vi "Test Get Right Menu on Card Inserted.vi"(8 "error in (no error)":errorcluster, 11 "Test Case In":refnum<class "View Model Test.lvclass">) -> (0 "error out":errorcluster, 3 "Test Case Out":refnum<class "View Model Test.lvclass">)   [LabVIEW 2020, in "View Model Test.lvclass"]
uses:
  View Model Test.lvclass
  View Model Test.lvclass/View Model Test.ctl
  01074fa8-ee8a-411d-bc8b-fc92c4f90959.vi
  ATM View Model/ATM View Model.lvclass
  ATM Controller/State.ctl
  ATM Controller/ATM Controller.lvclass
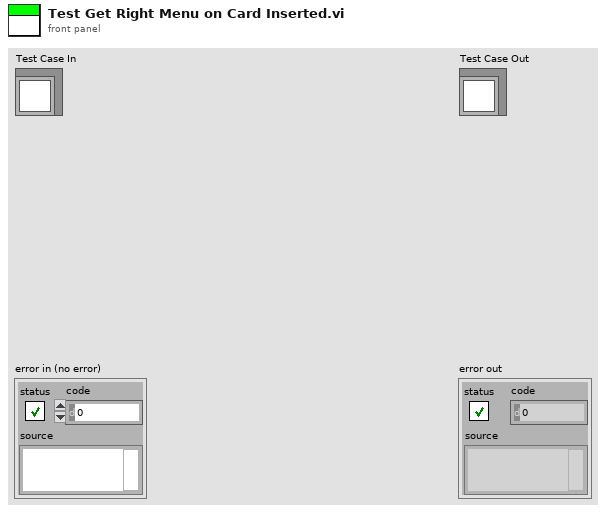
[diagram p1: front panel]
types:
  T1 = cluster{"RFS String":string, "RFS String 2":string, "RFS String 3":string}
  T2 = typedef "ATM Controller.lvclass/State.ctl" = enum16{"Start", "Card Inserted", "Verification Failed", "Verification Succeeded", "Depositing", "Depositing Completed", "Withdrawing", "Withdraw Completed", "Withdraw Failed", "Balance Inquiry", "Terminate"}
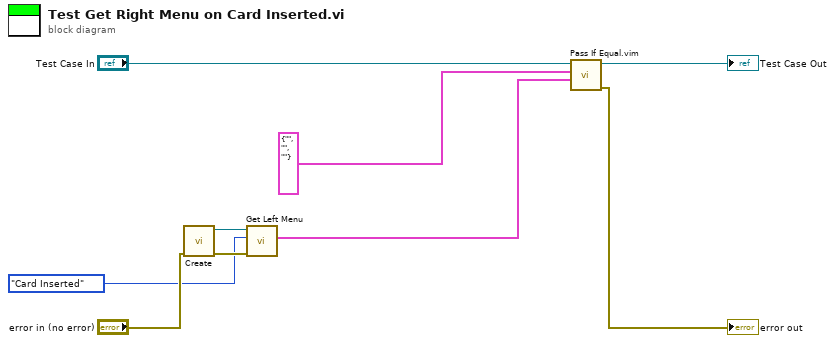
[diagram p0: block diagram]
diagram:
  n1 = call "Create.vi"("error in (no error)"="error in (no error)") -> ("error out"=w4:errorcluster, "ATM View Model out"=w5:refnum<class "ATM View Model.lvclass">)  [unwired: 9 in]
  n2 = call "Get Left Menu.vi"("error in (no error)"=w4, "ATM State"=State."Card Inserted", "ATM View Model in"=w5) -> ("Left Menu"=w3:T1)  [unwired: 6 in, 2 out]
  n3 = call "Pass If Equal.vim"("Actual"=w3, "Expected"=T1 {"RFS String"="", "RFS String 2"="", "RFS String 3"=""} ("Left Menu"), "LUnit Test Case In"="Test Case In") -> ("error out"=→"error out":errorcluster, "LUnit Test Case Out"=→"Test Case Out":refnum<class "View Model Test.lvclass">)  [unwired: 7 in]
